vi "test_Set Instrument Addon Name To Existing Name.vi"(8 "error in (no error)":errorcluster, 11 "TestCase in":refnum<class "Instrument Addon Scripting API Custom Device Unit Tests.lvclass">) -> (0 "error out":errorcluster, 3 "TestCase out":refnum<class "Instrument Addon Scripting API Custom Device Unit Tests.lvclass">)   [LabVIEW 2018, in "Instrument Addon Scripting API Custom Device Unit Tests.lvclass"]
uses:
  Instrument Addon Scripting API Custom Device Unit Tests.lvclass
  <vilib>/addons/_JKI Toolkits/VI Tester/TestCase.llb/TestCase.lvclass
  Instrument Addon Scripting API Test Assets/Instrument Addon Scripting API Test Assets.lvclass
  APIs/Scripting API/Instrument Addon Scripting API.lvlib
  C:/Program Files (x86)/National Instruments/LabVIEW 2018/vi.lib/addons/_JKI Toolkits/VI Tester/TestCase.llb/TestCase.lvclass
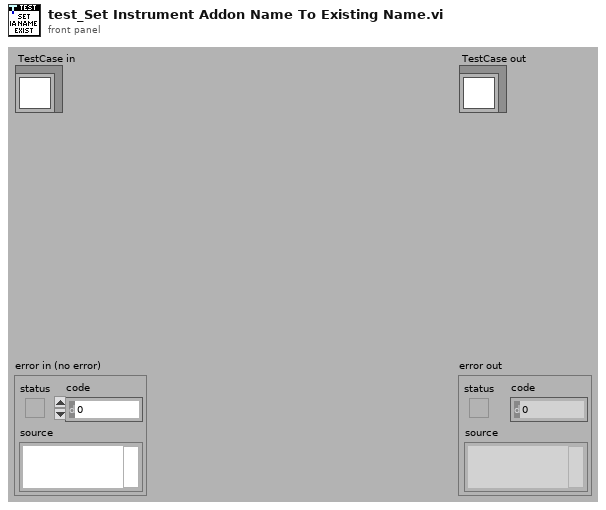
[diagram p1: front panel]
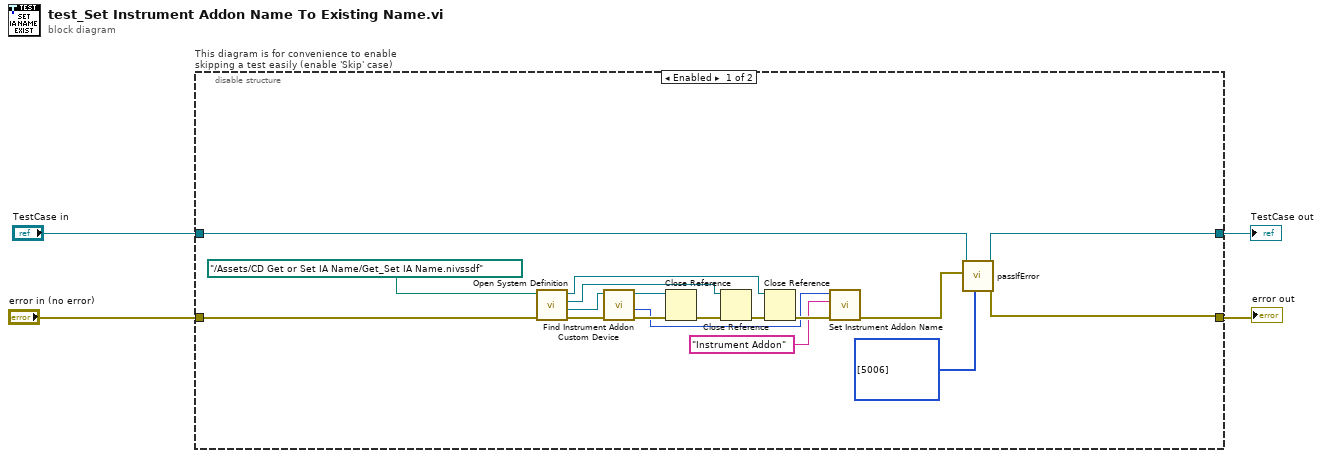
[diagram p0: block diagram]
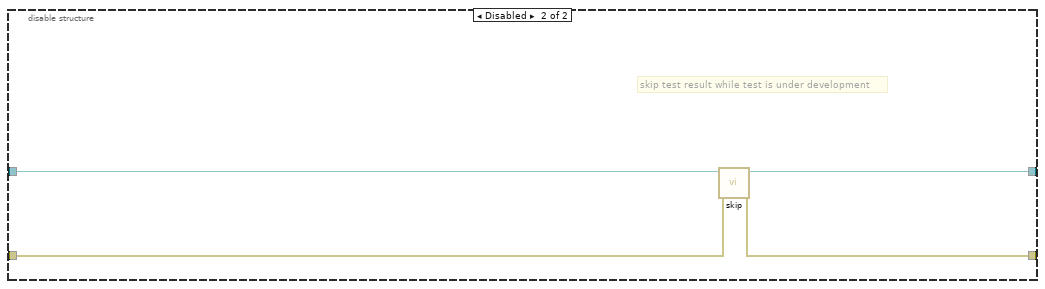
[diagram p2: hidden frame]
diagram:
  n1 = disable-structure "This diagram is for convenience to enable skipping a test easily (enable 'Skip' case)" shown="Enabled" {
    disable-tunnel: "TestCase in" -> [w22 w26]
    disable-tunnel: [w21 w24] -> w1
    disable-tunnel: [w20 w25] -> w3
    disable-tunnel: "error in (no error)" -> [w19 w23]
    frame Enabled {
      n2 = call "Open System Definition.vi"("error in (no error)"=w19, "System Definition File"=path "../Assets/CD Get or Set IA Name/Get_Set IA Name.nivssdf") -> ("error out"=w18:errorcluster, "Target Refnum"=w17:refnum<k24>, "Root Refnum"=w13:refnum<k24>, "System Definition Refnum"=w14:refnum<k24>)  [unwired: 6 in]
      n3 = call "Find Instrument Addon Custom Device.vi"("error in"=w18, "target in"=w17) -> ("error out"=w10:errorcluster, "NodeID"=w8:u64, "target out"=w11:refnum<k24>)  [unwired: 7 in]
      n4 = Close Reference(reference=w11, error in (no error)=w10) -> (error out=w12:errorcluster)
      n5 = Close Reference(reference=w13, error in (no error)=w12) -> (error out=w15:errorcluster)
      n6 = Close Reference(reference=w14, error in (no error)=w15) -> (error out=w9:errorcluster)
      n7 = call "Set Instrument Addon Name.vi"("Error In"=w9, "Name"="Instrument Addon", "Instrument Addon Refnum In"=w8) -> ("Error Out"=w6:errorcluster)  [unwired: 7 in, 1 out]
      n8 = call-dynamic "passIfError.vi"("passing error codes (default = any error code)"=i32[] [5006], "error"=w6, "TestCase in"=w22) -> ("error out"=w20:errorcluster, "TestCase out"=w21:refnum<class "Instrument Addon Scripting API Custom Device Unit Tests.lvclass">)  [unwired: 7 in]
    }
    frame Disabled {
      # "skip test result while test is under development"
      n9 = call <vilib>:"skip.vi"("error in (no error)"=w23, "TestCase in"=w26) -> ("error out"=w25:errorcluster, "TestCase out"=w24:refnum<class "Instrument Addon Scripting API Custom Device Unit Tests.lvclass">)  [unwired: 8 in]
    }
  }
  "error out" <- w3
  "TestCase out" <- w1
